vi "VCM_Check_Queue.vi"(7 "Error In":errorcluster caption="Fehler (Eingang)", 10 "queue":refnum<queue>) -> (0 "Error Out":errorcluster caption="Fehler (Ausgang)", 1 "VCM Control":T1, 3 "New Entries?":bool)   [LabVIEW 2019]
uses:
  Mischer/VCM-Control.ctl
panel:
  out "Numeric":dbl
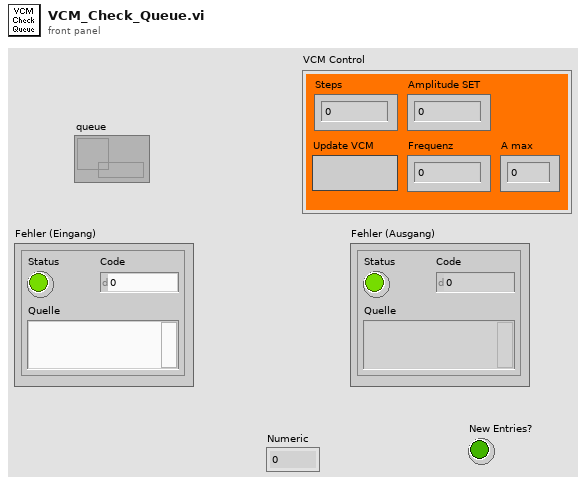
[diagram p1: front panel]
types:
  T1 = typedef "VCM-Control.ctl" = cluster{"Steps":dbl, "Amplitude SET":dbl, "Frequenz":dbl, "A max":dbl, "Update VCM":bool}
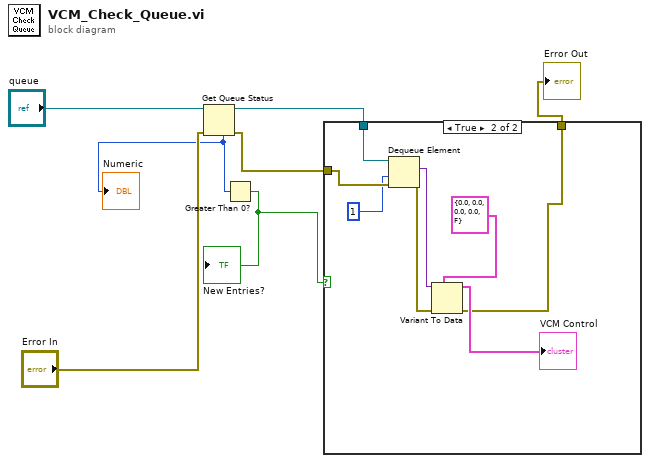
[diagram p0: block diagram]
diagram:
  n1 = Get Queue Status(queue="queue", error in (no error)="Error In") -> (queue out=w6:refnum<queue>, error out=w2:errorcluster, # elements in queue=w4:i32)  [unwired: 1 in, 5 out]
  "Numeric" <- w4
  n2 = Greater Than 0?(x=w4) -> (x > 0?=w3:bool)
  "New Entries?" <- w3
  n3 = case shown="True" w3 {
    tunnel: w6 -> [_ w16]
    tunnel: w2 -> [w8 w15]
    tunnel: [w8 w11] -> w1
    frame False {
    }
    frame True {
      n4 = Dequeue Element(queue=w16, timeout in ms (-1)=1, error in (no error)=w15) -> (element=w9:variant, error out=w13:errorcluster)  [unwired: 2 out]
      n5 = Variant To Data(error in=w13, type=T1 {"Steps"=0.0, "Amplitude SET"=0.0, "Frequenz"=0.0, "A max"=0.0, "Update VCM"=FALSE} ("VCM Control 2"), Variant=w9) -> (data=→"VCM Control":T1, error out=w11:errorcluster)
    }
  }
  "Error Out" <- w1
